vi "SplashScreen.vi"() -> ()   [LabVIEW 2019, in "GameEngine.lvlib"]
uses:
  GameEngine.lvlib
  <vilib>/Platform/TimedLoop/XDataNode/wakeup.ctl
  <vilib>/Platform/TimedLoop/XDataNode/XDNodeRunTimeDep.lvlib
  <vilib>/Platform/TimedLoop/XDataNode/nitl_modes.ctl
  <vilib>/Platform/TimedLoop/XDataNode/timing_clust.ctl
  <vilib>/platform/TimedLoop/XDataNode/XDataNode.xnode
  VGA/VGA.lvlib
  <vilib>/eio/EIONode/EIONode.xnode
  <vilib>/rvi/eio/common/nirviEmuTemplateMethod_errors.vi
  VGA/data.ctl
panel:
  in  "faderate (ticks)":u32=2000000
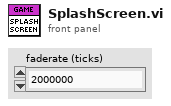
[diagram p1: front panel]
types:
  T1 = typedef "VGA.lvlib/data.ctl" = cluster{"x_frontporch":u8, "x_syncpulse":u8, "x_backporch":u8, "y_frontporch":u8, "y_syncpulse":u8, "y_backporch":u8, "DrawPixel?":bool, "x_tickcount":u16, "y_tickcount":u16, "x_Index":i16, "y_Index":i16}
  T2 = typedef "XDNodeRunTimeDep.lvlib/timing_clust.ctl" = cluster{"Expected End [f-1]":u64, "Actual End [f-1]":u64, "Finished Late? [f-1]":bool, "Expected End [i-1]":u64, "Actual End [i-1]":u64, "Finished Late? [i-1]":bool, "Expected Start [i]":u64, "Actual Start [i]":u64, "Expected Start [f]":u64, "Actual Start [f]":u64, "Source Name":string, "Structure Name":string, "Period":i64, "Deadline":i64, "Offset":i64, "Start":i64, "Priority":i32, "Timeout":i32, "Mode":T3, "Wakeup Reason":T4, "Error":errorcluster, "Source Type":string, "Secondary Source Type":string, "Global End Time":u64, "Global Start Time":u64, "Frame Duration":u64, "Iteration Duration":u64, "Assigned CPU":i32, "I/O Scan Engine Mode":u32}
  T3 = typedef "XDNodeRunTimeDep.lvlib/nitl_modes.ctl" = enum32{"No Change", "Process missed periods, maintain original phase", "Discard missed periods, maintain original phase", "Process missed periods, ignore original phase", "Discard missed periods, ignore original phase"}
  T4 = typedef "XDNodeRunTimeDep.lvlib/wakeup.ctl" = enum32{"Normal", "Aborted", "Asynchronous wakeup", "Timing source error", "Timed loop error", "Timeout"}
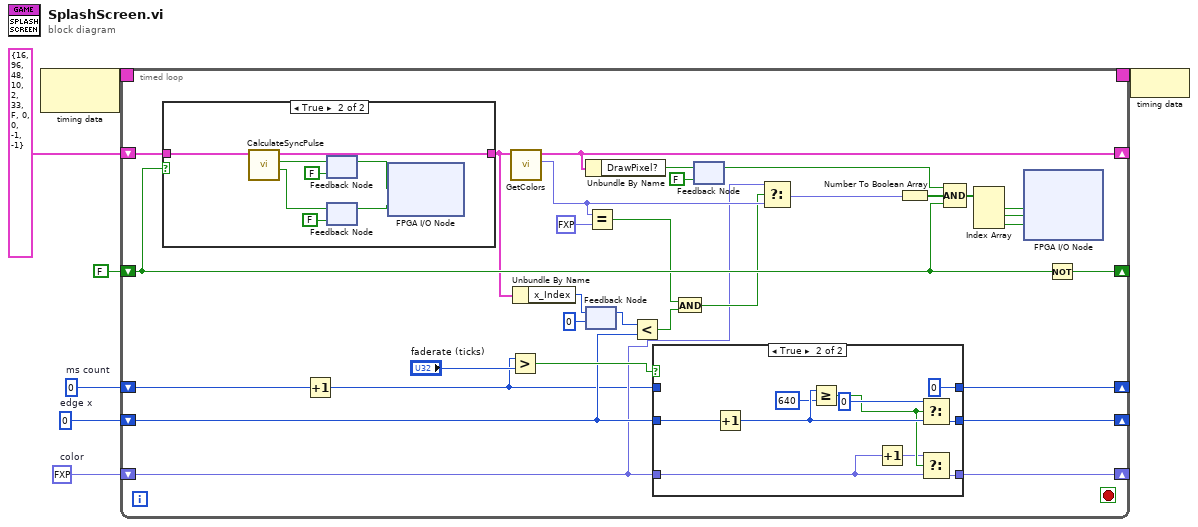
[diagram p0: block diagram]
diagram:
  w1 = fxp<+,3,3> 2.0  # color
  w2 = u16 0  # edge x
  w3 = u32 0  # ms count
  n1 = node-c288() -> (w7:T2)  [unwired: 1 in]
  n2 = timed-loop {
    timing: w7 -> [_]
    timing-out: [_] -> w6
    shift-right: [w33] -> _
    shift-left: T1 {"x_frontporch"=16, "x_syncpulse"=96, "x_backporch"=48, "y_frontporch"=10, "y_syncpulse"=2, "y_backporch"=33, "DrawPixel?"=FALSE, "x_tickcount"=0, "y_tickcount"=0, "x_Index"=-1, "y_Index"=-1} ("VGA_data") -> [w38]
    shift-right: [w36] -> _
    shift-left: FALSE -> [w34]
    shift-right: [w24] -> _
    shift-left: w3 -> [w11]
    shift-right: [w23] -> _
    shift-left: w2 -> [w20]
    shift-right: [w19] -> _
    shift-left: w1 -> [w12]
    stop <- _ stop-if-true
    n3 = case shown="True" w34 {
      tunnel: w38 -> [w52 w60]
      tunnel: [w52 w59] -> w26
      frame False {
      }
      frame True {
        n4 = call "CalculateSyncPulse.vi"("VGA_data"=w60) -> ("vSync"=w58:bool, "hSync"=w57:bool, "VGA_data 2"=w59:T1)  [unwired: 8 in]
        n5 = feedback-in #1(w57) -> ()
        n6 = feedback #1(FALSE ("hSync")) -> (w56:bool)
        n7 = feedback-in #2(w58) -> ()
        n8 = feedback #2(FALSE ("vSync")) -> (w55:bool)
        n9 = xnode "FPGA I/O Node"("hSync"=w56, "vSync"=w55) -> ()  [unwired: 2 in, 2 out]
      }
    }
    n10 = Increment(x=w11) -> (x+1=w10:u32)
    n11 = Greater?(x=w10, y="faderate (ticks)") -> (0:w22:bool)
    n12 = call "GetColors.vi"("VGA_data"=w26) -> ("Colors"=w18:fxp<+,3,3>, "VGA_data 2"=w33:T1)  [unwired: 9 in]
    n13 = Unbundle By Name(w26) -> ("x_Index"=w21:i16)
    n14 = Unbundle By Name(w33) -> ("DrawPixel?"=w32:bool)
    n15 = feedback-in #3(w21) -> ()
    n16 = feedback #3(i16 0 ("x_Index")) -> (w9:i16)
    n17 = Equal?(x=w18, y=fxp<+,3,3> 7.0) -> (x = y?=w15:bool)
    n18 = Less?(x=w9, y=w20) -> (x < y?=w16:bool)
    n19 = case shown="True" w22 {
      tunnel: w20 -> [w40 w51]
      tunnel: w10 -> [w41 _]
      tunnel: [w41 u32 0] -> w24
      tunnel: [w40 w47] -> w23
      tunnel: w12 -> [w39 w44]
      tunnel: [w39 w45] -> w19
      frame False {
      }
      frame True {
        n20 = Increment(x=w51) -> (x+1=w49:u16)
        n21 = Greater Or Equal?(x=w49, y=u16 640) -> (x >= y?=w43:bool)
        n22 = Increment(x=w44) -> (x+1=w42:fxp<+,3,3>)
        n23 = Select(t=u16 0, s=w43, f=w49) -> (s? t:f=w47:u16)
        n24 = Select(t=w42, s=w43, f=w44) -> (s? t:f=w45:fxp<+,3,3>)
      }
    }
    n25 = And(x=w15, y=w16) -> (x .and. y?=w13:bool)
    n26 = feedback #4(FALSE ("DrawPixel?")) -> (w28:bool)
    n27 = feedback-in #4(w32) -> ()
    n28 = Select(t=w12, s=w13, f=w18) -> (s? t:f=w14:fxp<+,3,3>)
    n29 = Number To Boolean Array(number=w14) -> (Boolean array=w37:bool[])
    n30 = Compound Arithmetic op=AND(w28, w37, w34) -> (w35:bool[])
    n31 = Index Array(array=w35) -> (element #1=w31:bool, element #2=w30:bool, element #3=w29:bool)  [unwired: 3 in]
    n32 = xnode "FPGA I/O Node"("RED"=w31, "GREEN"=w30, "BLUE"=w29) -> ()  [unwired: 3 in, 3 out]
    n33 = Not(x=w34) -> (.not. x?=w36:bool)
  }
  n34 = node-c288(w6) -> ()
